vi "ADC_Scan_Count.vi"(0 "pretrigger scans (0)":u32, 2 "post trigger scans (1000)":u32=1000, 3 "error in (no error)":errorcluster, 4 "number of channels":i32) -> (7 "Scan count string":string, 9 "error out":errorcluster)   [LabVIEW 2010]
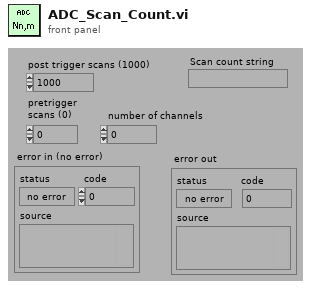
[diagram p1: front panel]
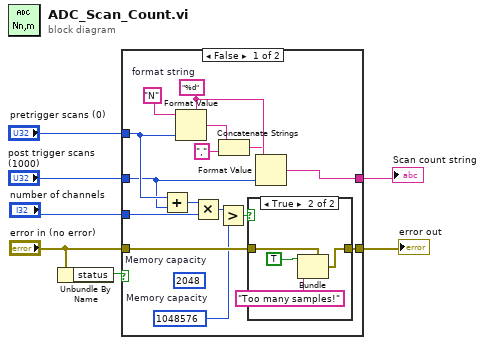
[diagram p0: block diagram]
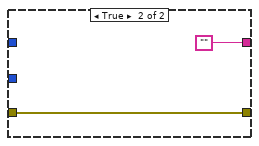
[diagram p3: hidden frame]
diagram:
  n1 = Unbundle By Name("error in (no error)") -> ("status"=w3:bool)
  n2 = case shown="False" w3 {
    tunnel: [w21 ""] -> w5
    tunnel: "post trigger scans (1000)" -> [w15 _]
    tunnel: "pretrigger scans (0)" -> [w16 _]
    tunnel: "error in (no error)" -> [w10 w29]
    tunnel: [w9 w29] -> w4
    tunnel: "number of channels" -> [w13 _]
    frame False {
      (unwired) u32 2048  # Memory capacity
      w8 = u32 1048576  # Memory capacity
      w22 = "%d"  # format string
      n3 = Add(x=w16, y=w15) -> (x+y=w14:u32)
      n4 = Format Value(string ("")="N", format string=w22, value (0)=w16) -> (output string=w18:string)
      n5 = Multiply(x=w14, y=w13) -> (x*y=w12:u32)
      n6 = Greater?(x=w12, y=w8) -> (0:w11:bool)
      n7 = Concatenate Strings(w18, ",") -> (w19:string)
      n8 = case shown="True" w11 {
        tunnel: w10 -> [w23 w27]
        tunnel: [w23 w26] -> w9
        frame False {
        }
        frame True {
          n9 = Bundle(cluster=w27, "status"=TRUE, "source"="Too many samples!") -> (w26:errorcluster)  [unwired: 1 out]
        }
      }
      n10 = Format Value(string ("")=w19, format string=w22, value (0)=w15) -> (output string=w21:string)
    }
    frame True {
    }
  }
  "Scan count string" <- w5
  "error out" <- w4
